vi "XNET Database Undeploy.vi"(0 "IP address":string, 5 "alias":string, 11 "error in (no error)":errorcluster) -> (15 "error out":errorcluster)   [LabVIEW 2018]
doc: "Undeploys a database from a remote LabVIEW Real-Time (RT) target."
uses:
  nixlvapi.dll
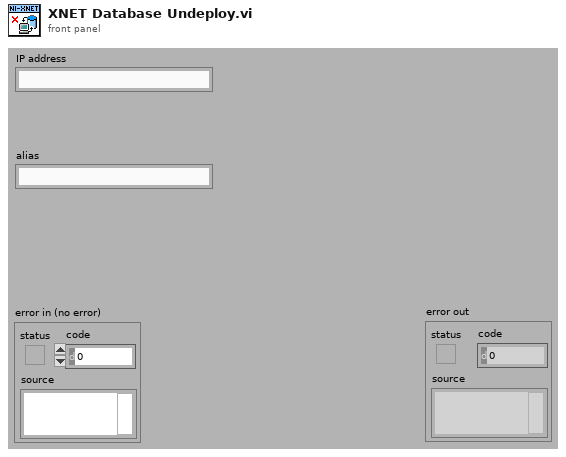
[diagram p1: front panel]
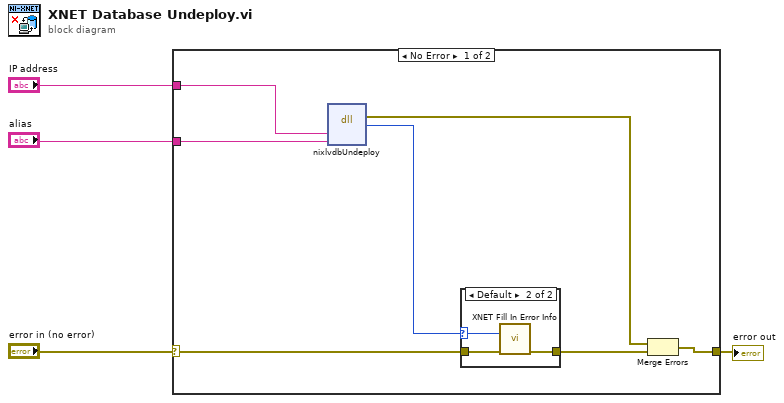
[diagram p0: block diagram]
diagram:
  n1 = case shown="No Error" "error in (no error)" {
    selector: "error in (no error)" -> [w10 w16]
    tunnel: "alias" -> [w8 _]
    tunnel: [w6 w16] -> w4
    tunnel: "IP address" -> [w7 _]
    frame No Error {
      n2 = dll-call lib="nixlvapi.*" fn="nixlvdbUndeploy" ("nilvxaiu.dll:lvxenDatabaseDeleteObject")("IPAddress"=w7, "DatabaseAlias"=w8) -> (error out=w5:errorcluster, "return type"=w9:i32)  [unwired: 5 in, 1 out]
      n3 = case shown="Default" w9 {
        selector: w9 -> [_ w13]
        tunnel: w10 -> [w12 w14]
        tunnel: [w12 w15] -> w11
        frame 0 {
        }
        frame Default {
          n4 = call "XNET Fill In Error Info.vi"("status code"=w13, "error in"=w14) -> ("error out"=w15:errorcluster)  [unwired: 13 out]
        }
      }
      n5 = Merge Errors(w5, w11) -> (w6:errorcluster)
    }
    frame Error {
    }
  }
  "error out" <- w4
